vi "ClientNTTestUpdate.vi"(8 "NT Connection":bool, 11 "TestConfig":T1) -> (0 "Value3":dbl, 1 "Value2":dbl, 2 "Value1":dbl, 3 "Value0":dbl, 4 "Good2":bool, 5 "Good1":bool, 6 "Good3":bool, 7 "Good0":bool)   [LabVIEW 2019]
uses:
  ClientNTTestConfig.ctl
  <vilib>/Rock Robotics/Network Tables/NT Read Number.vi
  <vilib>/Rock Robotics/WPI/ThirdParty/JAS_Junk/TrajLib/Util_GetTime.vi
  <vilib>/Rock Robotics/Network Tables/NT Write Number.vi
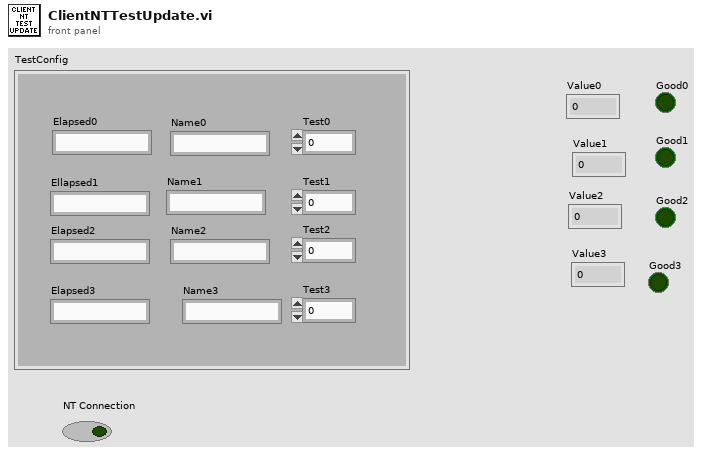
[diagram p1: front panel]
types:
  T1 = typedef "ClientNTTestConfig.ctl" = cluster{"Elapsed0":string, "Name0":string, "Test0":u32, "Ellapsed1":string, "Name1":string, "Test1":u32, "Elapsed2":string, "Name2":string, "Test2":u32, "Elapsed3":string, "Name3":string, "Test3":u32}
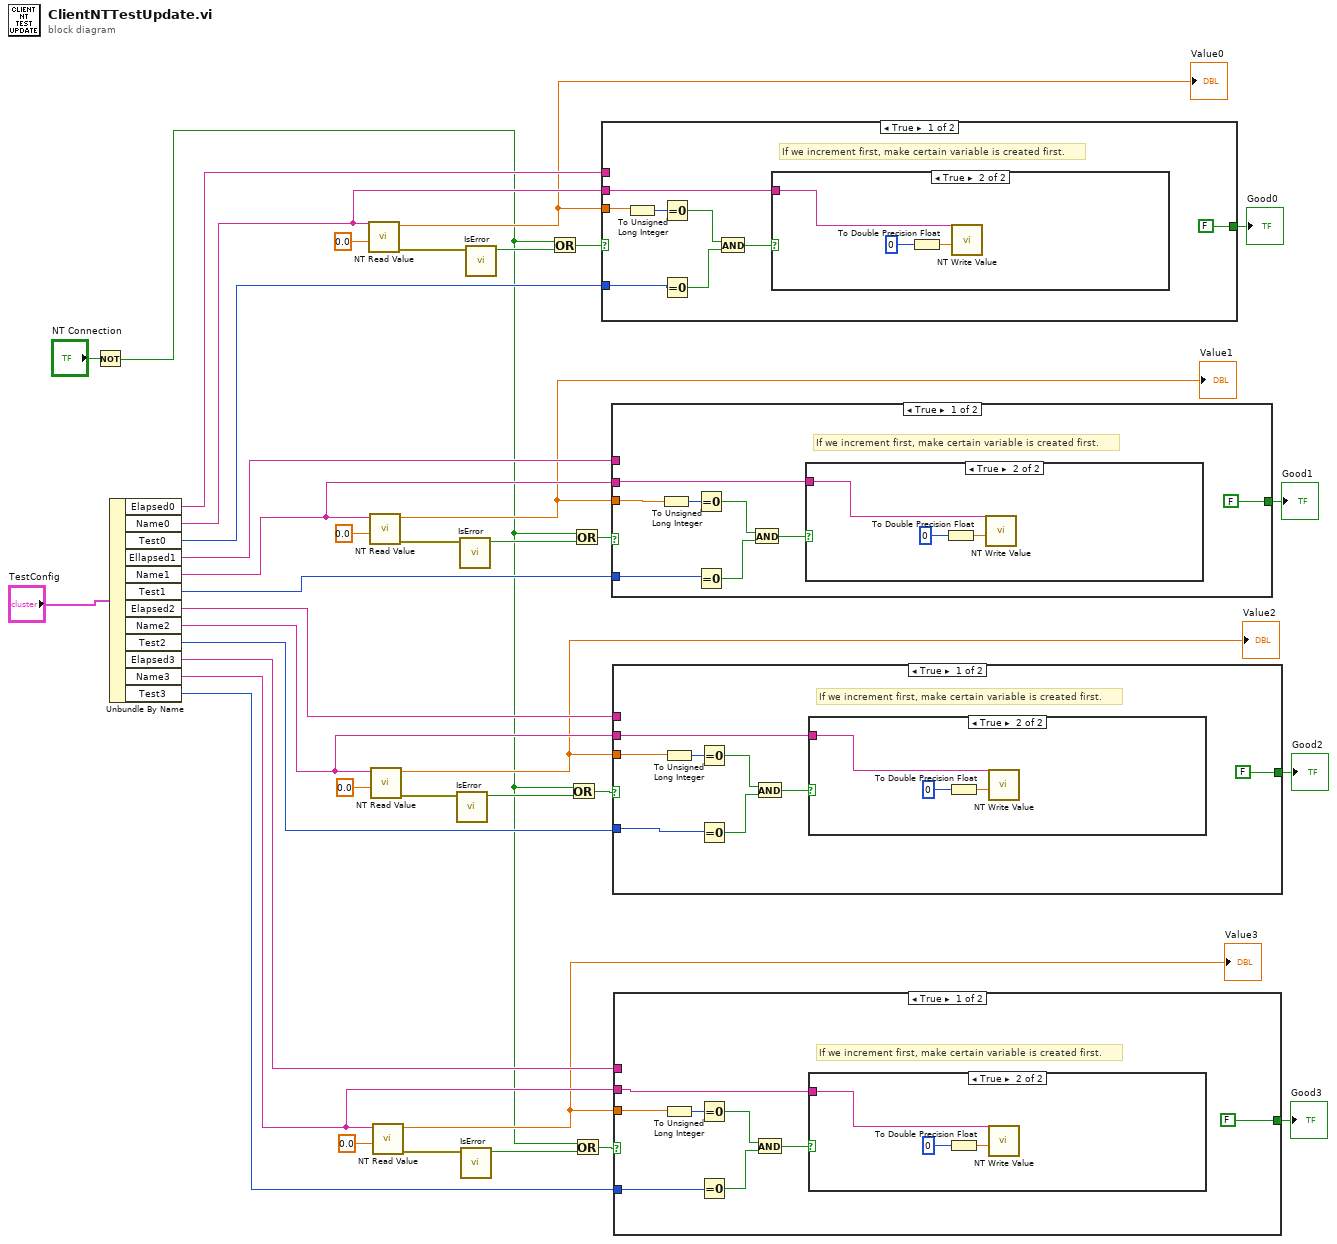
[diagram p0: block diagram]
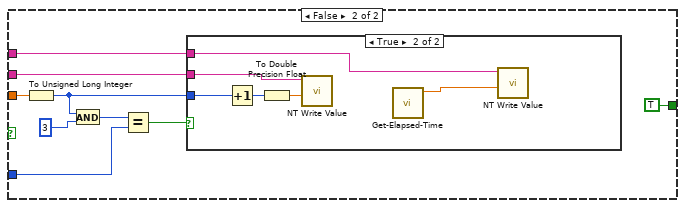
[diagram p3: hidden frame]
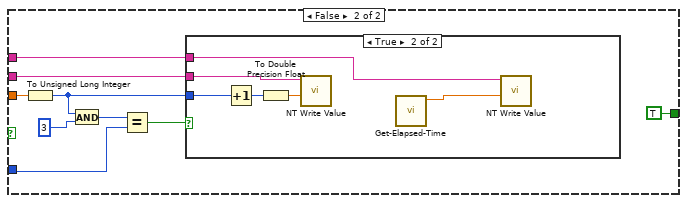
[diagram p6: hidden frame]
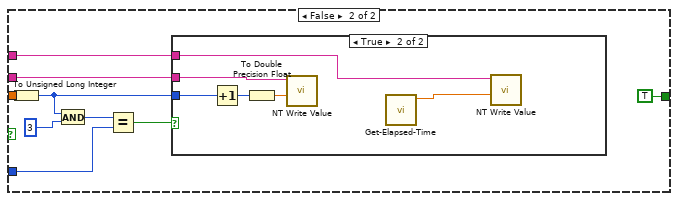
[diagram p9: hidden frame]
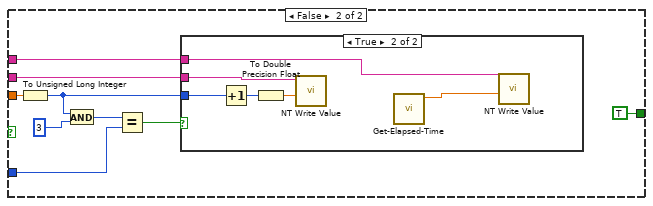
[diagram p12: hidden frame]
diagram:
  n1 = Not(x="NT Connection") -> (.not. x?=w1:bool)
  n2 = Unbundle By Name("TestConfig") -> ("Elapsed0"=w34:string, "Name0"=w33:string, "Test0"=w32:u32, "Ellapsed1"=w31:string, "Name1"=w30:string, "Test1"=w29:u32, "Elapsed2"=w28:string, "Name2"=w27:string, "Test2"=w26:u32, "Elapsed3"=w25:string, "Name3"=w24:string, "Test3"=w23:u32)
  n3 = call-poly <vilib>:"NT Read Value.vi"("Default Value"=0.0, "Name"=w33) -> ("error out"=w10:errorcluster, "Numeric"=w19:dbl)  [unwired: 8 in]
  "Value0" <- w19
  n4 = call-poly <vilib>:"NT Read Value.vi"("Default Value"=0.0, "Name"=w30) -> ("error out"=w12:errorcluster, "Numeric"=w22:dbl)  [unwired: 8 in]
  "Value1" <- w22
  n5 = call-poly <vilib>:"NT Read Value.vi"("Default Value"=0.0, "Name"=w27) -> ("error out"=w3:errorcluster, "Numeric"=w21:dbl)  [unwired: 8 in]
  "Value2" <- w21
  n6 = call-poly <vilib>:"NT Read Value.vi"("Default Value"=0.0, "Name"=w24) -> ("error out"=w5:errorcluster, "Numeric"=w20:dbl)  [unwired: 8 in]
  "Value3" <- w20
  n7 = call "IsError.vi"("error in (no error)"=w3) -> ("Boolean"=w7:bool)  [unwired: 10 in]
  n8 = call "IsError.vi"("error in (no error)"=w12) -> ("Boolean"=w11:bool)  [unwired: 10 in]
  n9 = call "IsError.vi"("error in (no error)"=w5) -> ("Boolean"=w6:bool)  [unwired: 10 in]
  n10 = call "IsError.vi"("error in (no error)"=w10) -> ("Boolean"=w9:bool)  [unwired: 10 in]
  n11 = Or(x=w1, y=w9) -> (x .or. y?=w8:bool)
  n12 = Or(x=w1, y=w7) -> (x .or. y?=w2:bool)
  n13 = Or(x=w1, y=w11) -> (x .or. y?=w13:bool)
  n14 = Or(x=w1, y=w6) -> (x .or. y?=w4:bool)
  n15 = case shown="True" w8 {
    tunnel: w34 -> [_ w55]
    tunnel: w33 -> [w41 w54]
    tunnel: w32 -> [w45 w53]
    tunnel: w19 -> [w47 w52]
    tunnel: [FALSE TRUE] -> w18
    frame True {
      # "If we increment first, make certain variable is created first."
      n16 = To Unsigned Long Integer(number=w47) -> (unsigned 32bit integer=w46:u32)
      n17 = Equal To 0?(x=w46) -> (x = 0?=w44:bool)
      n18 = Equal To 0?(x=w45) -> (x = 0?=w43:bool)
      n19 = And(x=w44, y=w43) -> (x .and. y?=w42:bool)
      n20 = case shown="True" w42 {
        tunnel: w41 -> [_ w48]
        frame False {
        }
        frame True {
          n21 = To Double Precision Float(number=u32 0) -> (double precision float=w50:dbl)
          n22 = call-poly <vilib>:"NT Write Value.vi"("Numeric"=w50, "Name"=w48) -> ()  [unwired: 9 in, 1 out]
        }
      }
    }
    frame False {
      n23 = To Unsigned Long Integer(number=w52) -> (unsigned 32bit integer=w58:u32)
      n24 = And(x=w58, y=u32 3) -> (x .and. y?=w59:u32)
      n25 = Equal?(x=w59, y=w53) -> (x = y?=w56:bool)
      n26 = case shown="True" w56 {
        tunnel: w54 -> [_ w64]
        tunnel: w58 -> [_ w65]
        tunnel: w55 -> [_ w60]
        frame False {
        }
        frame True {
          n27 = Increment(x=w65) -> (x+1=w62:u32)
          n28 = To Double Precision Float(number=w62) -> (double precision float=w61:dbl)
          n29 = call-poly <vilib>:"NT Write Value.vi"("Numeric"=w61, "Name"=w64) -> ()  [unwired: 9 in, 1 out]
          n30 = call "Get-Elapsed-Time.vi"() -> ("ElapsedTime"=w63:dbl)  [unwired: 11 in]
          n31 = call-poly <vilib>:"NT Write Value.vi"("Numeric"=w63, "Name"=w60) -> ()  [unwired: 9 in, 1 out]
        }
      }
    }
  }
  "Good0" <- w18
  n32 = case shown="True" w13 {
    tunnel: w31 -> [_ w81]
    tunnel: w30 -> [w69 w80]
    tunnel: w29 -> [w67 w79]
    tunnel: w22 -> [w68 w78]
    tunnel: [FALSE TRUE] -> w17
    frame True {
      # "If we increment first, make certain variable is created first."
      n33 = To Unsigned Long Integer(number=w68) -> (unsigned 32bit integer=w73:u32)
      n34 = Equal To 0?(x=w73) -> (x = 0?=w72:bool)
      n35 = Equal To 0?(x=w67) -> (x = 0?=w71:bool)
      n36 = And(x=w72, y=w71) -> (x .and. y?=w70:bool)
      n37 = case shown="True" w70 {
        tunnel: w69 -> [_ w74]
        frame False {
        }
        frame True {
          n38 = To Double Precision Float(number=u32 0) -> (double precision float=w76:dbl)
          n39 = call-poly <vilib>:"NT Write Value.vi"("Numeric"=w76, "Name"=w74) -> ()  [unwired: 9 in, 1 out]
        }
      }
    }
    frame False {
      n40 = To Unsigned Long Integer(number=w78) -> (unsigned 32bit integer=w84:u32)
      n41 = And(x=w84, y=u32 3) -> (x .and. y?=w85:u32)
      n42 = Equal?(x=w85, y=w79) -> (x = y?=w82:bool)
      n43 = case shown="True" w82 {
        tunnel: w80 -> [_ w90]
        tunnel: w84 -> [_ w91]
        tunnel: w81 -> [_ w86]
        frame False {
        }
        frame True {
          n44 = Increment(x=w91) -> (x+1=w88:u32)
          n45 = To Double Precision Float(number=w88) -> (double precision float=w87:dbl)
          n46 = call-poly <vilib>:"NT Write Value.vi"("Numeric"=w87, "Name"=w90) -> ()  [unwired: 9 in, 1 out]
          n47 = call "Get-Elapsed-Time.vi"() -> ("ElapsedTime"=w89:dbl)  [unwired: 11 in]
          n48 = call-poly <vilib>:"NT Write Value.vi"("Numeric"=w89, "Name"=w86) -> ()  [unwired: 9 in, 1 out]
        }
      }
    }
  }
  "Good1" <- w17
  n49 = case shown="True" w2 {
    tunnel: w28 -> [_ w107]
    tunnel: w27 -> [w93 w106]
    tunnel: w26 -> [w95 w105]
    tunnel: w21 -> [w94 w104]
    tunnel: [FALSE TRUE] -> w16
    frame True {
      # "If we increment first, make certain variable is created first."
      n50 = To Unsigned Long Integer(number=w94) -> (unsigned 32bit integer=w99:u32)
      n51 = Equal To 0?(x=w99) -> (x = 0?=w98:bool)
      n52 = Equal To 0?(x=w95) -> (x = 0?=w97:bool)
      n53 = And(x=w98, y=w97) -> (x .and. y?=w96:bool)
      n54 = case shown="True" w96 {
        tunnel: w93 -> [_ w100]
        frame False {
        }
        frame True {
          n55 = To Double Precision Float(number=u32 0) -> (double precision float=w102:dbl)
          n56 = call-poly <vilib>:"NT Write Value.vi"("Numeric"=w102, "Name"=w100) -> ()  [unwired: 9 in, 1 out]
        }
      }
    }
    frame False {
      n57 = To Unsigned Long Integer(number=w104) -> (unsigned 32bit integer=w110:u32)
      n58 = And(x=w110, y=u32 3) -> (x .and. y?=w111:u32)
      n59 = Equal?(x=w111, y=w105) -> (x = y?=w108:bool)
      n60 = case shown="True" w108 {
        tunnel: w106 -> [_ w116]
        tunnel: w110 -> [_ w117]
        tunnel: w107 -> [_ w112]
        frame False {
        }
        frame True {
          n61 = Increment(x=w117) -> (x+1=w114:u32)
          n62 = To Double Precision Float(number=w114) -> (double precision float=w113:dbl)
          n63 = call-poly <vilib>:"NT Write Value.vi"("Numeric"=w113, "Name"=w116) -> ()  [unwired: 9 in, 1 out]
          n64 = call "Get-Elapsed-Time.vi"() -> ("ElapsedTime"=w115:dbl)  [unwired: 11 in]
          n65 = call-poly <vilib>:"NT Write Value.vi"("Numeric"=w115, "Name"=w112) -> ()  [unwired: 9 in, 1 out]
        }
      }
    }
  }
  "Good2" <- w16
  n66 = case shown="True" w4 {
    tunnel: w25 -> [_ w133]
    tunnel: w24 -> [w121 w132]
    tunnel: w23 -> [w119 w131]
    tunnel: w20 -> [w120 w130]
    tunnel: [FALSE TRUE] -> w15
    frame True {
      # "If we increment first, make certain variable is created first."
      n67 = To Unsigned Long Integer(number=w120) -> (unsigned 32bit integer=w125:u32)
      n68 = Equal To 0?(x=w125) -> (x = 0?=w124:bool)
      n69 = Equal To 0?(x=w119) -> (x = 0?=w123:bool)
      n70 = And(x=w124, y=w123) -> (x .and. y?=w122:bool)
      n71 = case shown="True" w122 {
        tunnel: w121 -> [_ w126]
        frame False {
        }
        frame True {
          n72 = To Double Precision Float(number=u32 0) -> (double precision float=w128:dbl)
          n73 = call-poly <vilib>:"NT Write Value.vi"("Numeric"=w128, "Name"=w126) -> ()  [unwired: 9 in, 1 out]
        }
      }
    }
    frame False {
      n74 = To Unsigned Long Integer(number=w130) -> (unsigned 32bit integer=w136:u32)
      n75 = And(x=w136, y=u32 3) -> (x .and. y?=w137:u32)
      n76 = Equal?(x=w137, y=w131) -> (x = y?=w134:bool)
      n77 = case shown="True" w134 {
        tunnel: w132 -> [_ w142]
        tunnel: w136 -> [_ w143]
        tunnel: w133 -> [_ w138]
        frame False {
        }
        frame True {
          n78 = Increment(x=w143) -> (x+1=w140:u32)
          n79 = To Double Precision Float(number=w140) -> (double precision float=w139:dbl)
          n80 = call-poly <vilib>:"NT Write Value.vi"("Numeric"=w139, "Name"=w142) -> ()  [unwired: 9 in, 1 out]
          n81 = call "Get-Elapsed-Time.vi"() -> ("ElapsedTime"=w141:dbl)  [unwired: 11 in]
          n82 = call-poly <vilib>:"NT Write Value.vi"("Numeric"=w141, "Name"=w138) -> ()  [unwired: 9 in, 1 out]
        }
      }
    }
  }
  "Good3" <- w15
